vi "LeCroy Wave Series Acquire Waveform In Loop.vi"() -> ()   [LabVIEW 2015]
doc: "This example shows how to use autosetup and acquire a waveform on a single channel for acquiring waveforms in a loop until stopped by user."
uses:
  Public/Data/Read Single Waveform.vi
  LeCroy Wave Series.lvlib
panel:
  in  "Reset?":bool
  in  "Perform Auto Setup?":bool
  in  "Timeout (10000 ms)":u32=10000
  in  "Source (0: Channel 1)":u16(ring) items=["Channel 1", "Channel 2", "Channel 3", "Channel 4", "Memory 1", "Memory 2", "Memory 3", "Memory 4", "Function 1", "Function 2", "Function 3", "Function 4", "Function 5", "Function 6", "Function 7", "Function 8"]
  in  "stop":bool
  out "Waveform Data":waveform(dbl)(graph)
  in  "VISA resource name":refnum<visa-resource-name>="VICP::129.175.100.26"
  # "(c) 2008 - 2012 NATIONAL INSTRUMENTS.  ALL RIGHTS RESERVED."
  # "Directions:\n\n1. Setup the scope to be able to successfully single trigger on a signal applied to the channel selected in the \"Source\" control,  or set Perform Auto Setup? to True to perform an autosetup. \n\n2. On this front panel, enter the VISA Resource name for your scope. (e.g. VICP::123.45.67.8 for TCP/IP, GPIB::5::INSTR for GPIB). Modify the timeout if necessary.\n\n3. For an initial test, set the Reset? and Perform Auto Setup? controls to True, and then run the VI to find the signal.  Leave both set to False for subsequent runs.  The scope's AUX OUT or Cal Out is a good test signal to use."
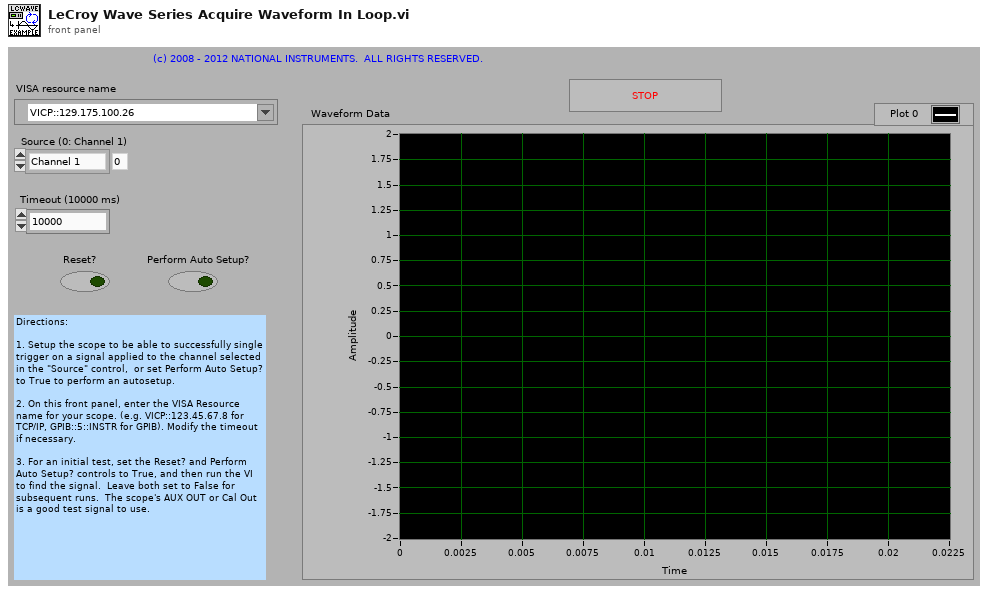
[diagram p1: front panel]
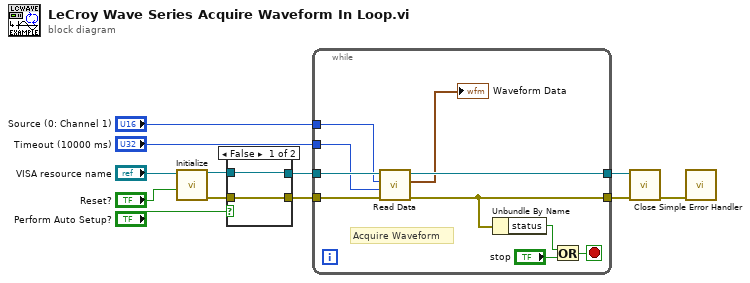
[diagram p0: block diagram]
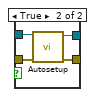
[diagram p2: hidden frame]
diagram:
  n1 = call "Initialize.vi"("Reset? (T: Yes)"="Reset?", "VISA resource name"="VISA resource name") -> ("error out"=w8:errorcluster, "VISA resource name out"=w7:refnum<visa-resource-name>)  [unwired: 8 in]
  n2 = case shown="False" "Perform Auto Setup?" {
    tunnel: w8 -> [w13 w18]
    tunnel: w7 -> [w14 w17]
    tunnel: [w14 w16] -> w6
    tunnel: [w13 w15] -> w5
    frame False {
    }
    frame True {
      n3 = call "Autosetup.vi"("error in (no error)"=w18, "VISA resource name"=w17) -> ("error out"=w15:errorcluster, "VISA resource name out"=w16:refnum<visa-resource-name>)  [unwired: 8 in]
    }
  }
  n4 = while {
    tunnel: w6 -> [w28]
    tunnel: w5 -> [w27]
    tunnel: [w26] -> w11
    tunnel: [w24] -> w10
    tunnel: "Source (0: Channel 1)" -> [w21]
    tunnel: "Timeout (10000 ms)" -> [w20]
    stop <- w25 stop-if-true
    # "Acquire Waveform"
    n5 = call-poly "Read Data.vi"("error in (no error)"=w27, "Timeout (10000 ms)"=w20, "Source (0: Channel 1)"=w21, "VISA resource name"=w28) -> ("error out"=w24:errorcluster, "Waveform Data"=→"Waveform Data":waveform(dbl), "VISA resource name out"=w26:refnum<visa-resource-name>)  [unwired: 5 in]
    n6 = Unbundle By Name(w24) -> ("status"=w23:bool)
    n7 = Or(x=w23, y="stop") -> (x .or. y?=w25:bool)
  }
  n8 = call "Close.vi"("error in (no error)"=w10, "VISA resource name"=w11) -> ("error out"=w12:errorcluster)  [unwired: 9 in]
  n9 = call <vilib>:"Simple Error Handler.vi"("error in (no error)"=w12) -> ()  [unwired: 4 in, 5 out]
